vi "Plot Prins FIFO Engine Result.vi"(6 "Plot Max Value":i32, 8 "error in (no error)":errorcluster, 9 "Number of Jobs":i32, 10 "Number of Machines":i32, 11 "FIFO Results":T1) -> (0 "error out":errorcluster, 3 "Graph Out":picture)   [LabVIEW 2013, in "Scheduler.lvclass"]
uses:
  Scheduler.lvclass
  Controls/Prins FIFO Scheduler Result Cluster.ctl
  <vilib>/Heliosphere Research LLC/Advanced Plotting Toolkit/typedefs/PlotColor.ctl
  <vilib>/Heliosphere Research LLC/Advanced Plotting Toolkit/api_figure/TicksProperties.ctl
  <vilib>/Heliosphere Research LLC/Advanced Plotting Toolkit/properties/Text.ctl
  <vilib>/Heliosphere Research LLC/Advanced Plotting Toolkit/properties/Text_FontSize.ctl
  <vilib>/Heliosphere Research LLC/Advanced Plotting Toolkit/properties/Text_FontStyle.ctl
  <vilib>/Heliosphere Research LLC/Advanced Plotting Toolkit/api_annotations/ShapeProperties.ctl
  <vilib>/Heliosphere Research LLC/Advanced Plotting Toolkit/properties/Line.ctl
  <vilib>/Heliosphere Research LLC/Advanced Plotting Toolkit/properties/Line_Style.ctl
  <vilib>/Heliosphere Research LLC/Advanced Plotting Toolkit/properties/Display.ctl
  <vilib>/Heliosphere Research LLC/Advanced Plotting Toolkit/api_annotations/TextProperties.ctl
  <vilib>/Heliosphere Research LLC/Advanced Plotting Toolkit/Advanced Plotting Toolkit.lvlib
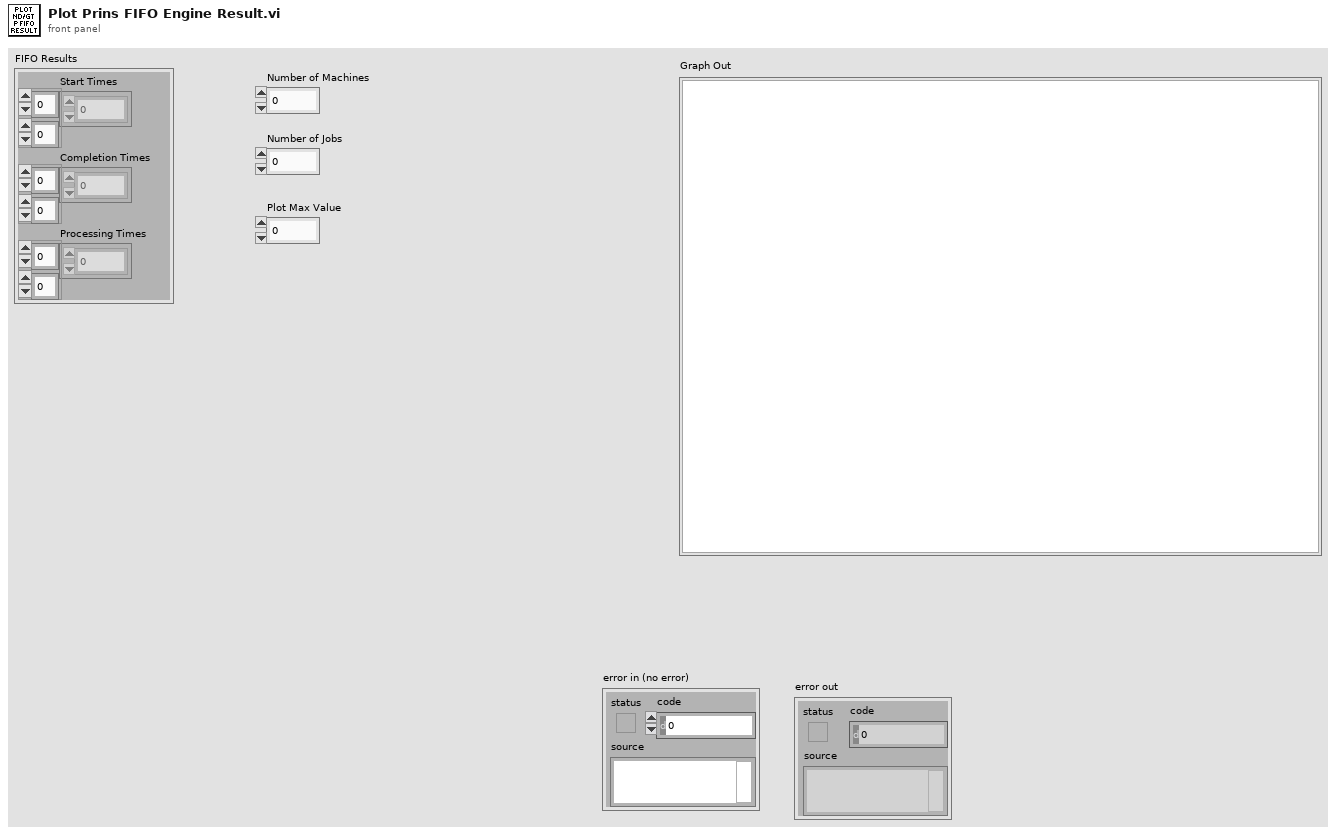
[diagram p1: front panel]
types:
  T1 = typedef "Scheduler.lvclass/Prins FIFO Scheduler Result Cluster.ctl" = cluster{"Start Times":u16[][], "Completion Times":u16[][], "Processing Times":u16[][]}
  T2 = typedef "Advanced Plotting Toolkit.lvlib/Text_FontSize.ctl" = i32
  T3 = typedef "Advanced Plotting Toolkit.lvlib/TicksProperties.ctl" = cluster{"Text":T4}
  T4 = typedef "Advanced Plotting Toolkit.lvlib/Text.ctl" = cluster{"Color":T5, "Background Color":T5, "Font Size (points)":T2, "Font Style":T6, "Rotation Angle":dbl}
  T5 = typedef "Advanced Plotting Toolkit.lvlib/PlotColor.ctl" = u32
  T6 = typedef "Advanced Plotting Toolkit.lvlib/Text_FontStyle.ctl" = enum16{"Automatic", "Normal", "Italic", "Bold"}
  T7 = typedef "Advanced Plotting Toolkit.lvlib/PlotID.ctl" = i32
  T8 = typedef "Advanced Plotting Toolkit.lvlib/TextProperties.ctl" = cluster{"Text":T4, "Display":T9}
  T9 = typedef "Advanced Plotting Toolkit.lvlib/Display.ctl" = cluster{"Alpha":dbl, "Z Order":dbl}
  T10 = typedef "Advanced Plotting Toolkit.lvlib/ShapeProperties.ctl" = cluster{"Color":T5, "Line":T11, "Display":T9}
  T11 = typedef "Advanced Plotting Toolkit.lvlib/Line.ctl" = cluster{"Style":T12, "Color":T5, "Width":sgl}
  T12 = typedef "Advanced Plotting Toolkit.lvlib/Line_Style.ctl" = enum16{"Automatic", "Solid", "Dashed", "Dotted", "Dash-dot", "Invisible"}
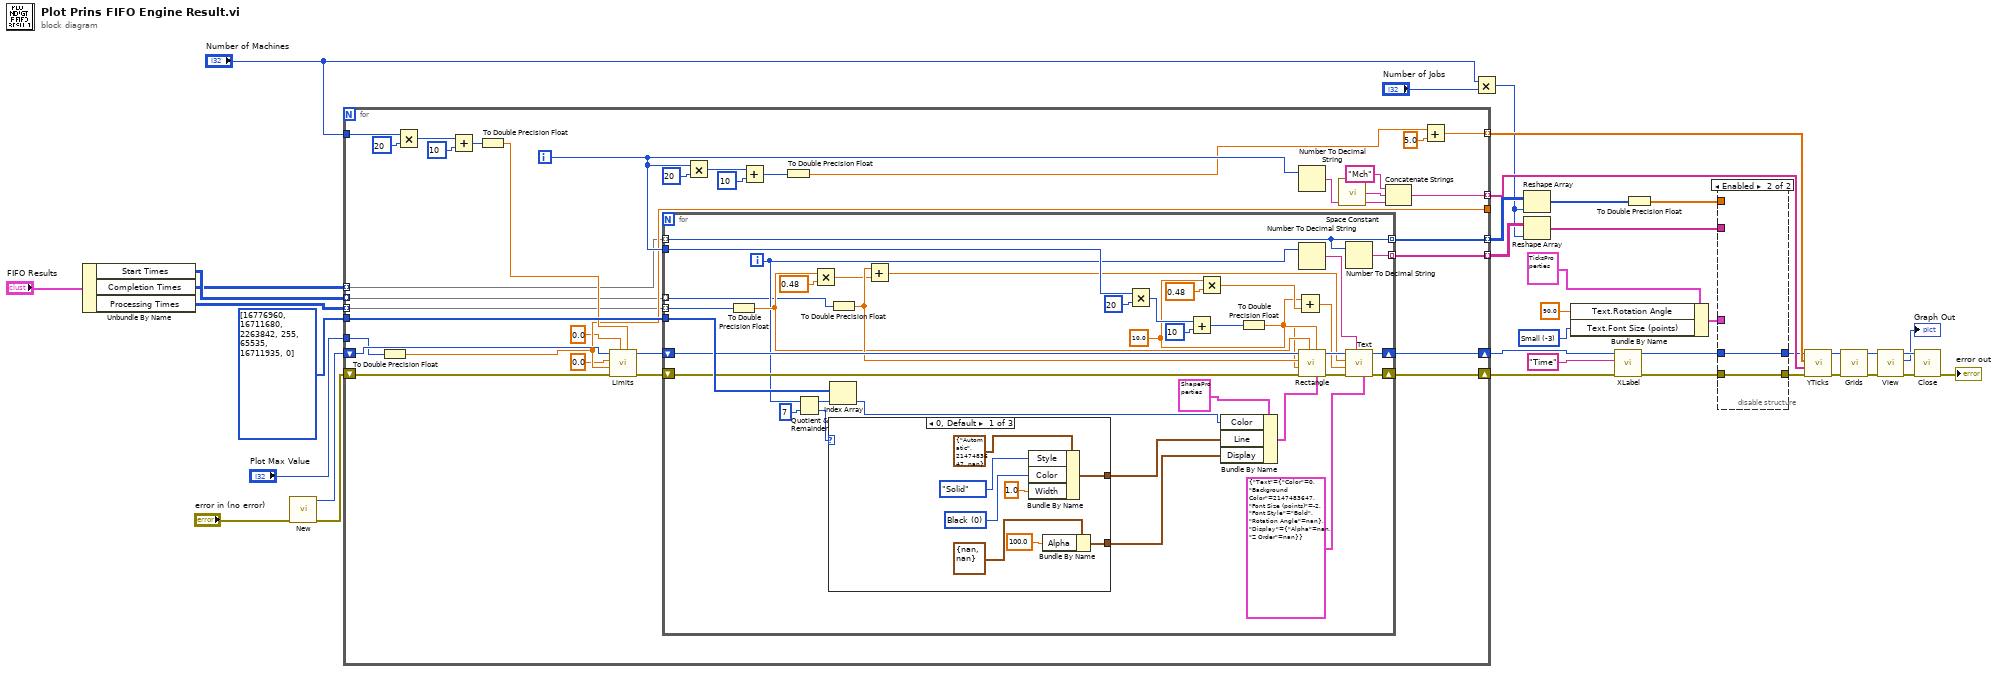
[diagram p0: block diagram]
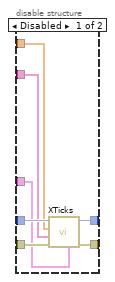
[diagram p2: hidden frame]
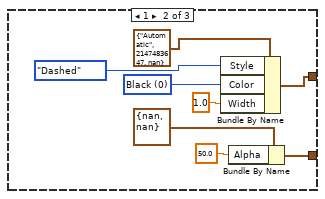
[diagram p3: hidden frame]
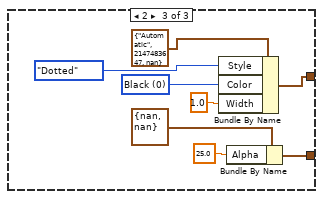
[diagram p4: hidden frame]
diagram:
  w12 = T2 -3 items=["Automatic"=0, "XX-Small"=-1, "X-Small"=-2, "Small"=-3, "Medium"=-4, "Large"=-5, "X-Large"=-6, "XX-Large"=-7] ("Text.Font Size (points)")
  w33 = T5[] [16776960, 16711680, 2263842, 255, 65535, 16711935, 0] items=["Automatic"=2147483647, "Black"=0, "White"=16777215, "Red"=16711680, "Green"=2263842, "Blue"=255, "Cyan"=65535, "Magenta"=16711935, "Yellow"=16776960]
  n1 = Unbundle By Name("FIFO Results") -> ("Start Times"=w5:u16[][], "Completion Times"=w4:u16[][], "Processing Times"=w3:u16[][])
  n2 = call <vilib>:"New.vi"("error in (no error)"="error in (no error)") -> ("error out"=w34:errorcluster, "Plot ID"=w35:T7)  [unwired: 9 in]
  n3 = for {
    shift-right: [w72] -> w31
    shift-left: w34 -> [w69]
    shift-right: [w71] -> w32
    shift-left: w35 -> [w67]
    tunnel: w33 -> [w70]
    tunnel: [w59] -> w25 mode=indexing
    tunnel: [w49] -> w24 mode=indexing
    tunnel: [w48] -> w11 mode=indexing
    tunnel: [w47] -> w19 mode=indexing
    tunnel: [w46] -> _
    tunnel: "Number of Machines" -> [w45]
    tunnel: "Plot Max Value" -> [w44]
    tunnel: w5 -> [w41] mode=indexing
    tunnel: w4 -> [w40] mode=indexing
    tunnel: w3 -> [w39] mode=indexing
    i -> [w52]
    n4 = To Double Precision Float(number=w44) -> (double precision float=w46:dbl)
    n5 = Multiply(x=w45, y=20) -> (x*y=w65:i32)
    n6 = Add(x=w65, y=10) -> (x+y=w63:i32)
    n7 = To Double Precision Float(number=w63) -> (double precision float=w57:dbl)
    n8 = call <vilib>:"Limits.vi"("Y Max"=w57, "Y Min"=0.0, "error in (no error)"=w69, "X Max"=w46, "X Min"=0.0, "Plot ID"=w67) -> ("error out"=w68:errorcluster, "Plot ID Out"=w62:T7)  [unwired: 4 in]
    n9 = for {
      shift-right: [w89] -> w72
      shift-left: w68 -> [w108]
      shift-right: [w91] -> w71
      shift-left: w62 -> [w107]
      tunnel: w70 -> [w109]
      tunnel: w52 -> [w99]
      tunnel: [w73] -> w48 mode=indexing
      tunnel: [w93] -> w47 mode=indexing
      tunnel: w41 -> [w75] mode=indexing
      tunnel: w40 -> [w73] mode=indexing
      tunnel: w39 -> [w74] mode=indexing
      i -> [w76]
      w81 = 10.0 ("Height")
      n10 = To Double Precision Float(number=w74) -> (double precision float=w87:dbl)
      n11 = Quotient & Remainder(x=w76, y=7) -> (x-y*floor(x/y)=w96:i32, floor(x/y)=w95:i32)
      n12 = Multiply(x=w87, y=0.48) -> (x*y=w85:dbl)
      n13 = case shown="0, Default" w95 {
        tunnel: [w113 w121 w129] -> w98
        tunnel: [w110 w118 w126] -> w94
        frame 0, Default {
          w115 = T5 0 items=["Automatic"=2147483647, "Black"=0, "White"=16777215, "Red"=16711680, "Green"=2263842, "Blue"=255, "Cyan"=65535, "Magenta"=16711935, "Yellow"=16776960] ("Color")
          n14 = Bundle By Name(cluster=T11 {"Style"=enum."Automatic", "Color"=2147483647, "Width"=nan} ("Line"), "Style"=Line_Style."Solid", "Color"=w115, "Width"=sgl 1.0) -> (w113:T11)
          n15 = Bundle By Name(cluster=T9 {"Alpha"=nan, "Z Order"=nan} ("Display"), "Alpha"=100.0) -> (w110:T9)
        }
        frame 1 {
          w123 = T5 0 items=["Automatic"=2147483647, "Black"=0, "White"=16777215, "Red"=16711680, "Green"=2263842, "Blue"=255, "Cyan"=65535, "Magenta"=16711935, "Yellow"=16776960] ("Color")
          n16 = Bundle By Name(cluster=T11 {"Style"=enum."Automatic", "Color"=2147483647, "Width"=nan} ("Line"), "Style"=Line_Style."Dashed", "Color"=w123, "Width"=sgl 1.0) -> (w121:T11)
          n17 = Bundle By Name(cluster=T9 {"Alpha"=nan, "Z Order"=nan} ("Display"), "Alpha"=50.0) -> (w118:T9)
        }
        frame 2 {
          w131 = T5 0 items=["Automatic"=2147483647, "Black"=0, "White"=16777215, "Red"=16711680, "Green"=2263842, "Blue"=255, "Cyan"=65535, "Magenta"=16711935, "Yellow"=16776960] ("Color")
          n18 = Bundle By Name(cluster=T11 {"Style"=enum."Automatic", "Color"=2147483647, "Width"=nan} ("Line"), "Style"=Line_Style."Dotted", "Color"=w131, "Width"=sgl 1.0) -> (w129:T11)
          n19 = Bundle By Name(cluster=T9 {"Alpha"=nan, "Z Order"=nan} ("Display"), "Alpha"=25.0) -> (w126:T9)
        }
      }
      n20 = Index Array(array=w109, index=w96) -> (element=w104:T5)
      n21 = To Double Precision Float(number=w75) -> (double precision float=w88:dbl)
      n22 = Add(x=w88, y=w85) -> (x+y=w84:dbl)
      n23 = Multiply(x=w99, y=20) -> (x*y=w102:i32)
      n24 = Add(x=w102, y=10) -> (x+y=w100:i32)
      n25 = Multiply(x=w81, y=0.48) -> (x*y=w83:dbl)
      n26 = Bundle By Name(cluster=T10 {"Color"=2147483647, "Line"={"Style"=enum."Automatic", "Color"=2147483647, "Width"=nan}, "Display"={"Alpha"=nan, "Z Order"=nan}} ("Properties"), "Color"=w104, "Line"=w98, "Display"=w94) -> (w105:T10)
      n27 = To Double Precision Float(number=w100) -> (double precision float=w80:dbl)
      n28 = Add(x=w80, y=w83) -> (x+y=w79:dbl)
      n29 = Number To Decimal String(number=w76) -> (decimal integer string=w78:string)  [unwired: 1 in]
      n30 = call <vilib>:"Rectangle.vi"("Properties"=w105, "Height"=w81, "Width"=w87, "error in (no error)"=w108, "Y Position"=w80, "X Position"=w88, "Plot ID"=w107) -> ("error out"=w90:errorcluster, "Plot ID Out"=w92:T7)  [unwired: 3 in]
      n31 = Number To Decimal String(number=w73) -> (decimal integer string=w93:string)  [unwired: 1 in]
      n32 = call <vilib>:"Text.vi"("Properties"=T8 {"Text"={"Color"=0, "Background Color"=2147483647, "Font Size (points)"=-2, "Font Style"=enum."Bold", "Rotation Angle"=nan}, "Display"={"Alpha"=nan, "Z Order"=nan}}, "Text"=w78, "error in (no error)"=w90, "Y Position"=w79, "X Position"=w84, "Plot ID"=w92) -> ("error out"=w89:errorcluster, "Plot ID Out"=w91:T7)  [unwired: 4 in]
    }
    n33 = Multiply(x=w52, y=20) -> (x*y=w55:i32)
    n34 = Add(x=w55, y=10) -> (x+y=w53:i32)
    n35 = To Double Precision Float(number=w53) -> (double precision float=w51:dbl)
    n36 = Number To Decimal String(number=w52) -> (decimal integer string=w58:string)  [unwired: 1 in]
    n37 = call <vilib>:"Space Constant.vi"() -> ("String"=w60:string)
    n38 = Concatenate Strings("Mch", w60, w58) -> (w59:string)
    n39 = Add(x=w51, y=5.0) -> (x+y=w49:dbl)
  }
  n40 = Multiply(x="Number of Machines", y="Number of Jobs") -> (x*y=w8:i32)
  n41 = Reshape Array(w11, w8) -> (w17:u16[])
  n42 = Reshape Array(w19, w8) -> (w18:string[])
  n43 = Bundle By Name(cluster=T3 {"Text"={"Color"=2147483647, "Background Color"=2147483647, "Font Size (points)"=0, "Font Style"=enum."Automatic", "Rotation Angle"=nan}} ("Properties"), "Text.Rotation Angle"=90.0, "Text.Font Size (points)"=w12) -> (w13:T3)
  n44 = call <vilib>:"XLabel.vi"("error in (no error)"=w31, "Label"="Time", "Plot ID"=w32) -> ("error out"=w21:errorcluster, "Plot ID out"=w23:T7)  [unwired: 7 in]
  n45 = To Double Precision Float(number=w17) -> (double precision float=w16:dbl[])
  n46 = disable-structure shown="Enabled" {
    disable-tunnel: w23 -> [w140 w142]
    disable-tunnel: [w139 w142] -> w22
    disable-tunnel: w21 -> [w138 w141]
    disable-tunnel: [w137 w141] -> w20
    disable-tunnel: w18 -> [w136 _]
    disable-tunnel: w16 -> [w135 _]
    disable-tunnel: w13 -> [w134 _]
    frame Disabled {
      n47 = call <vilib>:"XTicks.vi"("Properties"=w134, "error in (no error)"=w138, "Tick Labels"=w136, "Tick Locations"=w135, "Plot ID"=w140) -> ("error out"=w137:errorcluster, "Plot ID Out"=w139:T7)  [unwired: 5 in]
    }
    frame Enabled {
    }
  }
  n48 = call <vilib>:"YTicks.vi"("error in (no error)"=w20, "Tick Labels"=w25, "Tick Locations"=w24, "Plot ID"=w22) -> ("error out"=w27:errorcluster, "Plot ID Out"=w26:T7)  [unwired: 6 in]
  n49 = call <vilib>:"Grids.vi"("error in (no error)"=w27, "Plot ID"=w26) -> ("error out"=w30:errorcluster, "Plot ID Out"=w28:T7)  [unwired: 8 in]
  n50 = call <vilib>:"View.vi"("error in (no error)"=w30, "Plot ID"=w28) -> ("error out"=w9:errorcluster, "Picture"=→"Graph Out":picture, "Plot ID Out"=w10:T7)  [unwired: 7 in]
  n51 = call <vilib>:"Close.vi"("error in (no error)"=w9, "Plot ID"=w10) -> ("error out"=→"error out":errorcluster)  [unwired: 9 in]
